vi "poly_sub_filter_single_wav.vi"(6 "add info? (T)":bool=TRUE, 8 "error in (no error)":errorcluster, 9 "f":i32=50 caption="base frequency (50Hz)", 10 "N":i32=3 caption="N of harmonics to remove (3)", 11 "waveform in":waveform(dbl)) -> (0 "error out":errorcluster, 3 "waveform out":waveform(dbl))   [LabVIEW 2015]
uses:
  <vilib>/measure/matone.llb/Extract Single Tone Information 1 Chan.vi
  <vilib>/measure/NI_MAPro.lvlib
  <vilib>/Analysis/NI_AALBase.lvlib
panel:
  out "graph":cluster{dbl[], dbl[]}[](graph) caption="Automatic line filter level detection"
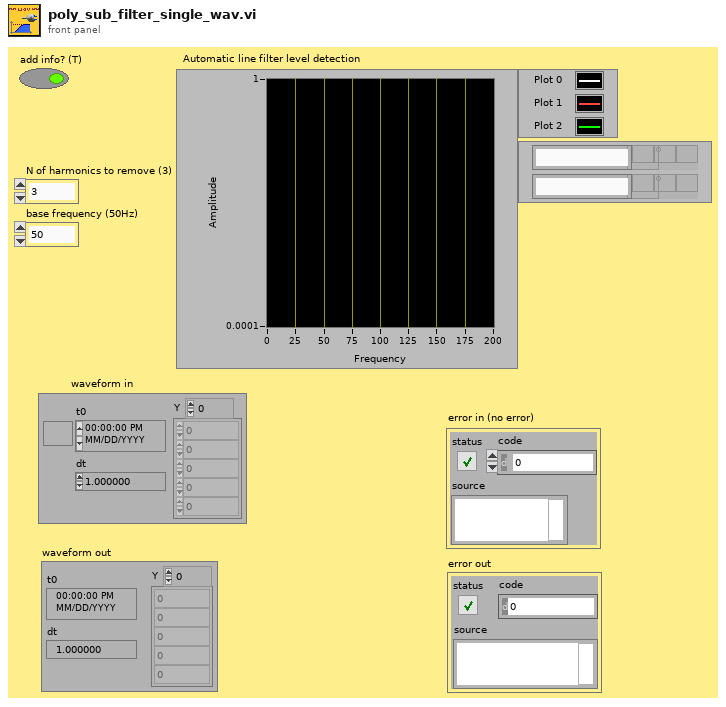
[diagram p1: front panel]
types:
  T1 = enum32{"none", "input signal", "detected signal", "residual signal"}
  T2 = cluster{"approx freq. (optional)":dbl, "search (+/- % of Fsampl.)":dbl}
  T3 = cluster{"exported time signal":waveform(dbl), "exported spectrum (dB)":cluster{"f0":dbl, "df":dbl, "dB Spectrum (Hann)":dbl[]}}
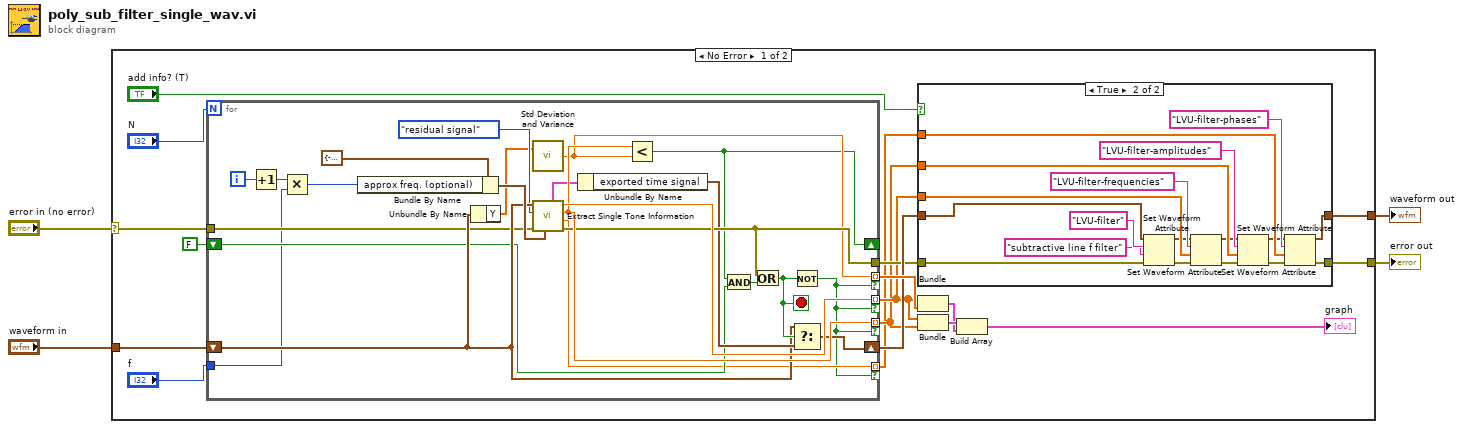
[diagram p0: block diagram]
diagram:
  n1 = case shown="No Error" "error in (no error)" {
    selector: "error in (no error)" -> [w16 w65]
    tunnel: [w6 w65] -> w4
    tunnel: "waveform in" -> [w13 w66]
    tunnel: [w7 w66] -> w1
    frame No Error {
      n2 = for {
        N: "N" -> [_]
        shift-right: [w56] -> w12
        shift-left: w13 -> [w53]
        tunnel: [w64] -> w10 mode=indexing if=w45
        tunnel: [w57] -> w11
        tunnel: [w58] -> w9 mode=indexing if=w45
        tunnel: [w52] -> w20 mode=indexing if=w45
        shift-right: [w50] -> _
        shift-left: FALSE -> [w51]
        tunnel: w16 -> [w48]
        tunnel: "f" -> [w47]
        tunnel: [w46] -> w8 mode=indexing if=w45
        i -> [w61]
        stop <- w55 stop-if-true
        n3 = Increment(x=w61) -> (x+1=w60:i32)
        n4 = Multiply(x=w60, y=w47) -> (x*y=w59:i32)
        n5 = Bundle By Name(cluster=T2 {"approx freq. (optional)"=-1.0, "search (+/- % of Fsampl.)"=5.0} ("advanced search"), "approx freq. (optional)"=w59) -> (w62:T2)
        n6 = Unbundle By Name(w53) -> ("Y"=w43:dbl[])
        n7 = call <vilib>:"Std Deviation and Variance.vi"("X"=w43) -> ("standard deviation"=w52:dbl)  [unwired: 1 in, 2 out]
        n8 = call-poly <vilib>:"Extract Single Tone Information.vi"("advanced search"=w62, "error in (no error)"=w48, "export mode"=T1."residual signal", "time signal in"=w53) -> ("error out"=w57:errorcluster, "detected phase (deg)"=w46:dbl, "detected amplitude"=w58:dbl, "detected frequency"=w64:dbl, "exported signals"=w42:T3)  [unwired: 2 in, 1 out]
        n9 = Unbundle By Name(w42) -> ("exported time signal"=w54:waveform(dbl))
        n10 = Less?(x=w58, y=w52) -> (x < y?=w50:bool)
        n11 = And(x=w50, y=w51) -> (x .and. y?=w49:bool)
        n12 = Or(x=w57, y=w49) -> (x .or. y?=w55:bool)
        n13 = Not(x=w55) -> (.not. x?=w45:bool)
        n14 = Select(t=w53, s=w55, f=w54) -> (s? t:f=w56:waveform(dbl))
      }
      n15 = case shown="True" "add info? (T)" {
        tunnel: w12 -> [w23 w41]
        tunnel: w11 -> [w22 w38]
        tunnel: w10 -> [_ w36]
        tunnel: w9 -> [_ w32]
        tunnel: w8 -> [_ w28]
        tunnel: [w23 w25] -> w7
        tunnel: [w22 w24] -> w6
        frame False {
        }
        frame True {
          n16 = Set Waveform Attribute(4:w38, 5:"subtractive line f filter" ("name"), 6:"LVU-filter" ("name"), 7:w41) -> (0:w34:errorcluster, 3:w35:waveform(dbl))  [unwired: 1 out]
          n17 = Set Waveform Attribute(4:w34, 5:w36, 6:"LVU-filter-frequencies" ("name"), 7:w35) -> (0:w30:errorcluster, 3:w31:waveform(dbl))  [unwired: 1 out]
          n18 = Set Waveform Attribute(4:w30, 5:w32, 6:"LVU-filter-amplitudes" ("name"), 7:w31) -> (0:w26:errorcluster, 3:w27:waveform(dbl))  [unwired: 1 out]
          n19 = Set Waveform Attribute(4:w26, 5:w28, 6:"LVU-filter-phases" ("name"), 7:w27) -> (0:w24:errorcluster, 3:w25:waveform(dbl))  [unwired: 1 out]
        }
      }
      n20 = Bundle(w10, w20) -> (w18:cluster{dbl[], dbl[]})  [unwired: 1 in]
      n21 = Bundle(w10, w9) -> (w19:cluster{dbl[], dbl[]})  [unwired: 1 in]
      n22 = Build Array(w19, w18) -> (→"graph":cluster{dbl[], dbl[]}[])
    }
    frame Error {
    }
  }
  "error out" <- w4
  "waveform out" <- w1
